vi "Start array.vi"(10 "Set voltage":i32=4500, 11 "Set time":i32=60) -> (3 "Start array":string[](array[string]))   [LabVIEW 2014]
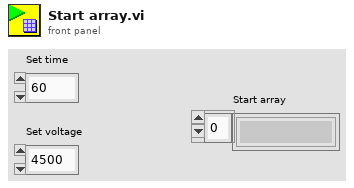
[diagram p1: front panel]
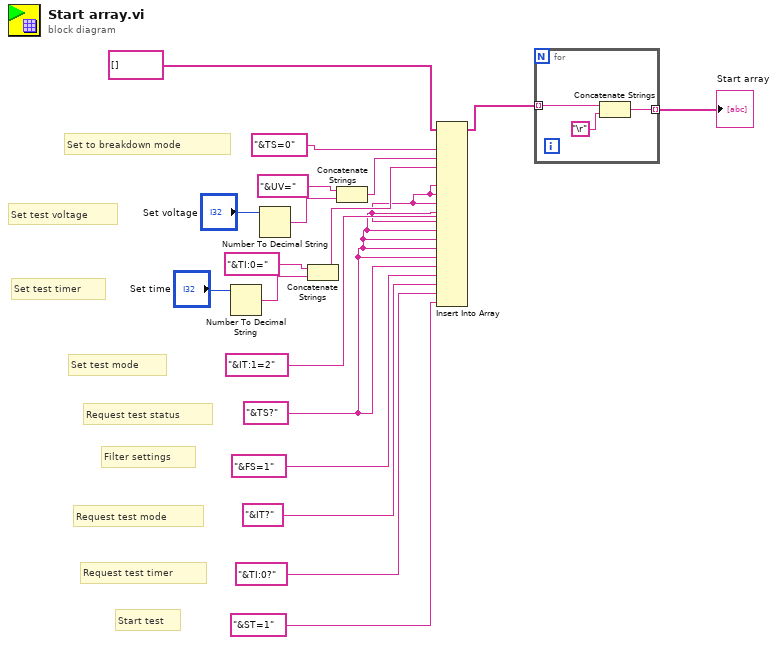
[diagram p0: block diagram]
diagram:
  w7 = "&TS?" ("write buffer")
  # "Request test timer"
  # "Set to breakdown mode"
  # "Request test mode"
  # "Start test"
  # "Filter settings"
  # "Request test status"
  # "Set test mode"
  # "Set test timer"
  # "Set test voltage"
  n1 = Number To Decimal String(number="Set time") -> (decimal integer string=w13:string)  [unwired: 1 in]
  n2 = Number To Decimal String(number="Set voltage") -> (decimal integer string=w17:string)  [unwired: 1 in]
  n3 = Concatenate Strings("&TI:0=" ("write buffer"), w13) -> (w11:string)
  n4 = Concatenate Strings("&UV=" ("write buffer"), w17) -> (w15:string)
  n5 = Insert Into Array(array=string[] [], new element #1="&TS=0" ("write buffer"), new element #2=w15, new element #3=w11, new element #4="&IT:1=2" ("write buffer"), new element #5=w7, new element #6=w7, new element #7=w7, new element #8=w7, new element #9=w7, new element #10=w7, new element #11=w7, new element #12=w7, new element #13=w7, new element #14=w7, new element #15="&FS=1" ("write buffer"), new element #16="&IT?" ("write buffer"), new element #17="&TI:0?" ("write buffer"), new element #18="&ST=1" ("write buffer")) -> (w9:string[])  [unwired: 1 in]
  n6 = for {
    tunnel: w9 -> [w20] mode=indexing
    tunnel: [w19] -> w3 mode=indexing
    n7 = Concatenate Strings(w20, "\r") -> (w19:string)
  }
  "Start array" <- w3
